vi "act-0026-01-cor.vi"() -> ()   [LabVIEW 2010]
panel:
  out "nb éléments tc":i32
  out "nb éléments dN(tc)":i32
  out "tc":dbl[](array[numeric])
  out "dN(tc)":u32[](array[numeric])
  out "tdeb":dbl[](array[numeric])
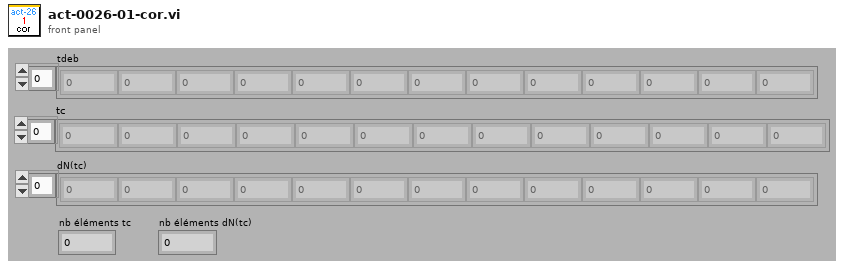
[diagram p1: front panel]
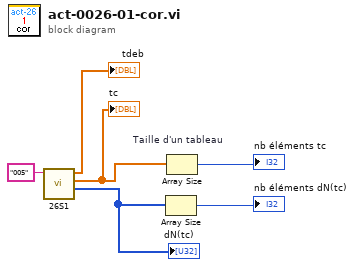
[diagram p0: block diagram]
diagram:
  n1 = call "26S1.vi"("src"="005") -> ("dN(tc)"=w1:u32[], "tc"=w2:dbl[], "tdeb"=→"tdeb":dbl[])  [unwired: 6 in, 2 out]
  "dN(tc)" <- w1
  "tc" <- w2
  n2 = Array Size(array=w1) -> (size(s)=→"nb éléments dN(tc)":i32)
  n3 = Array Size "Taille d'un tableau"(array=w2) -> (size(s)=→"nb éléments tc":i32)
